vi "Service Mode Entry.vi"(0 "GEA2 Reference In":refnum<k24>, 5 "Model":enum16{"HE", "LE"}(ring), 11 "Error In":errorcluster) -> (4 "GEA2 Reference Out":refnum<k24>, 6 "Pass/Fail?":bool, 8 "Report Text":string, 15 "Error Out":errorcluster)   [LabVIEW 2016, in "2015 VA Washer.lvlib"]
doc: "Use this VI to enter service mode."
uses:
  Projects/2015 VA Washer.lvlib
  C:/Automation/DLLs/PC Dot Net/GeaCommunication.dll
  Common/LabVIEW GEA2 Toolkit/LabVIEW_GEA2_Toolkit.lvlibp/type defs/Source_Destination.ctl
  Common/LabVIEW GEA2 Toolkit/LabVIEW_GEA2_Toolkit.lvlibp/type defs/ERD Read Data In.ctl
  Common/LabVIEW GEA2 Toolkit/LabVIEW_GEA2_Toolkit.lvlibp/type defs/Data Type.ctl
  type defs/Encoder Position.ctl
  Common/LabVIEW GEA2 Toolkit/LabVIEW_GEA2_Toolkit.lvlibp/type defs/ERD Write Data In.ctl
  Common/LabVIEW GEA2 Toolkit/LabVIEW_GEA2_Toolkit.lvlibp
panel:
  in  "Standalone?":bool
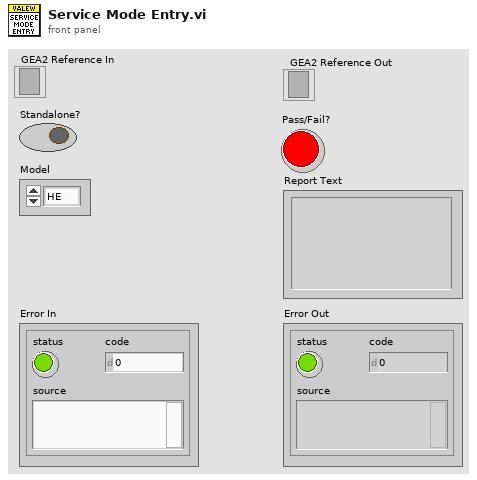
[diagram p1: front panel]
types:
  T1 = typedef "LabVIEW_GEA2_Toolkit.lvlibp/ERD Read Data In.ctl" = cluster{"ERD Number":u16, "Data Type":T2}
  T2 = typedef "LabVIEW_GEA2_Toolkit.lvlibp/Data Type.ctl" = enum16{"string", "boolean", "uint8_t", "uint16_t", "uint32_t", "uint64_t", "int8_t", "int16_t", "int32_t", "int64_t"}
  T3 = typedef "LabVIEW_GEA2_Toolkit.lvlibp/Source_Destination.ctl" = cluster{"Source":u8, "Destination":u8}
  T4 = typedef "LabVIEW_GEA2_Toolkit.lvlibp/ERD Write Data In.ctl" = cluster{"ERD Number":u16, "Data Type":T2, "Data":string}
  T5 = typedef "2015 VA Washer.lvlib/Encoder Position.ctl" = enum16{"Position 0", "Position 1", "Position 2", "Position 3", "Position 4", "Position 5", "Position 6", "Position 7", "Position 8", "Position 9", "Position 10", "Position 11", "Position 12", "Position 13", "Clear / Reset"}
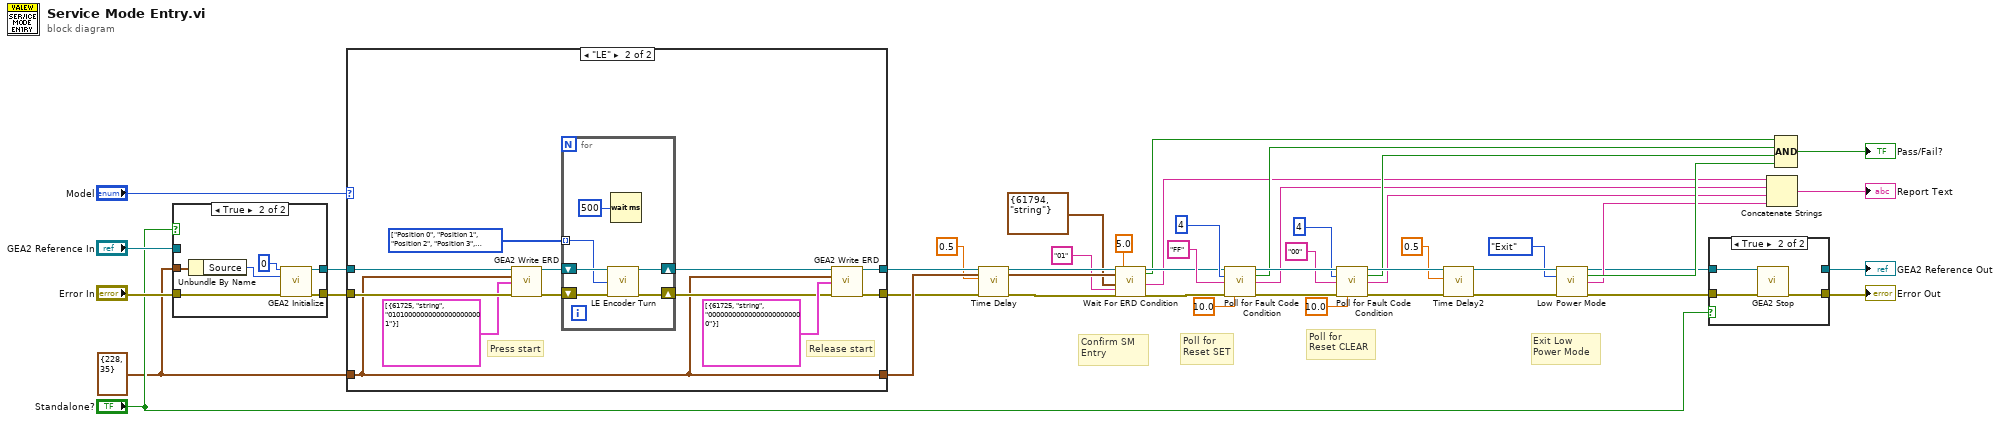
[diagram p0: block diagram]
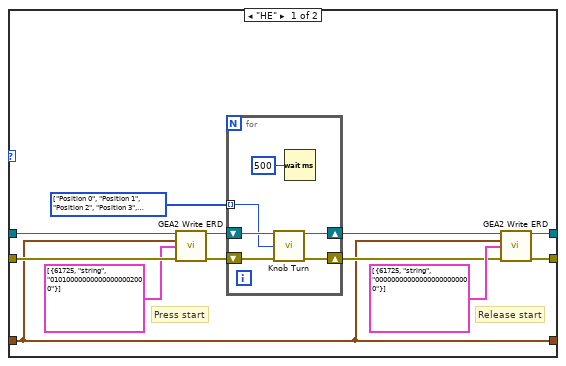
[diagram p2: hidden frame]
diagram:
  w37 = T3 {"Source"=228, "Destination"=35} ("GEA Inputs")
  # "Confirm SM \nEntry"
  # "Exit Low \nPower Mode"
  # "Poll for\nReset CLEAR"
  # "Poll for\nReset SET"
  n1 = case shown="True" "Standalone?" {
    tunnel: "Error In" -> [w45 w52]
    tunnel: [w45 w51] -> w39
    tunnel: "GEA2 Reference In" -> [w46 _]
    tunnel: [w46 w50] -> w40
    tunnel: w37 -> [_ w48]
    frame False {
    }
    frame True {
      n2 = Unbundle By Name(w48) -> ("Source"=w49:u8)
      n3 = call "GEA2 Initialize.vi"("Board Index"=0, "Source Address"=w49, "error in"=w52) -> ("GEA2 Reference Out"=w50:refnum<k24>, "error out"=w51:errorcluster)  [unwired: 10 in, 1 out]
    }
  }
  n4 = case shown="\"LE\"" "Model" {
    tunnel: w40 -> [w61 w79]
    tunnel: w39 -> [w60 w78]
    tunnel: w37 -> [w53 w71]
    tunnel: [w55 w73] -> w36
    tunnel: [w54 w72] -> w34
    tunnel: [w53 w71] -> w35
    frame "HE" {
      w64 = T5[] [enum."Position 0", enum."Position 1", enum."Position 2", enum."Position 3", enum."Position 4", enum."Position 5", enum."Position 6", enum."Position 7"] items=["Position 0", "Position 1", "Position 2", "Position 3", "Position 4", "Position 5", "Position 6", "Position 7", "Position 8", "Position 9", "Position 10", "Position 11", "Position 12", "Position 13", "Clear / Reset"]
      # "Release start"
      # "Press start"
      n5 = call "GEA2 Write ERD.vi"("GEA2 Reference In"=w61, "GEA Inputs"=w53, "Write ERD List"=T4[] [{"ERD Number"=61725, "Data Type"=enum."string", "Data"="010100000000000000002000"}], "Error In"=w60) -> ("GEA2 Reference Out"=w63:refnum<k24>, "Error Out"=w62:errorcluster)  [unwired: 9 in, 1 out]
      n6 = for {
        shift-right: [w69] -> w56
        shift-left: w63 -> [w70]
        shift-right: [w67] -> w57
        shift-left: w62 -> [w68]
        tunnel: w64 -> [w66] mode=indexing
        n7 = call "Knob Turn.vi"("GEA2 Reference In"=w70, "Button"=w66, "Error In"=w68) -> ("GEA2 Reference Out"=w69:refnum<k24>, "Error Out"=w67:errorcluster)  [unwired: 11 in]
        n8 = Wait (ms)(milliseconds to wait=u32 500) -> ()  [unwired: 1 out]
      }
      n9 = call "GEA2 Write ERD.vi"("GEA2 Reference In"=w56, "GEA Inputs"=w53, "Write ERD List"=T4[] [{"ERD Number"=61725, "Data Type"=enum."string", "Data"="000000000000000000000000"}], "Error In"=w57) -> ("GEA2 Reference Out"=w55:refnum<k24>, "Error Out"=w54:errorcluster)  [unwired: 9 in, 1 out]
    }
    frame "LE" {
      w82 = T5[] [enum."Position 0", enum."Position 1", enum."Position 2", enum."Position 3", enum."Position 4", enum."Position 5", enum."Position 6", enum."Position 7"] items=["Position 0", "Position 1", "Position 2", "Position 3", "Position 4", "Position 5", "Position 6", "Position 7", "Position 8", "Position 9", "Position 10", "Position 11", "Position 12", "Position 13", "Clear / Reset"]
      # "Release start"
      # "Press start"
      n10 = call "GEA2 Write ERD.vi"("GEA2 Reference In"=w79, "GEA Inputs"=w71, "Write ERD List"=T4[] [{"ERD Number"=61725, "Data Type"=enum."string", "Data"="010100000000000000000001"}], "Error In"=w78) -> ("GEA2 Reference Out"=w81:refnum<k24>, "Error Out"=w80:errorcluster)  [unwired: 9 in, 1 out]
      n11 = for {
        shift-right: [w87] -> w74
        shift-left: w81 -> [w88]
        shift-right: [w85] -> w75
        shift-left: w80 -> [w86]
        tunnel: w82 -> [w84] mode=indexing
        n12 = call "LE Encoder Turn.vi"("GEA2 Reference In"=w88, "Button"=w84, "Error In"=w86) -> ("GEA2 Reference Out"=w87:refnum<k24>, "Error Out"=w85:errorcluster)  [unwired: 11 in]
        n13 = Wait (ms)(milliseconds to wait=u32 500) -> ()  [unwired: 1 out]
      }
      n14 = call "GEA2 Write ERD.vi"("GEA2 Reference In"=w74, "GEA Inputs"=w71, "Write ERD List"=T4[] [{"ERD Number"=61725, "Data Type"=enum."string", "Data"="000000000000000000000000"}], "Error In"=w75) -> ("GEA2 Reference Out"=w73:refnum<k24>, "Error Out"=w72:errorcluster)  [unwired: 9 in, 1 out]
    }
  }
  n15 = call "Time Delay"("error in (no error)"=w34, "Delay Time (s)"=0.5) -> ("error out"=w5:errorcluster)  [unwired: 9 in]
  n16 = call "Wait For ERD Condition.vi"("GEA2 Reference In"=w36, "GEA Inputs"=w35, "ERD Read Data"=T1 {"ERD Number"=61794, "Data Type"=enum."string"} ("ERD Read Data In"), "Expected Low"="01", "Error In"=w5, "Timeout (s)"=5.0) -> ("GEA2 Reference Out"=w18:refnum<k24>, "Pass/Fail?"=w6:bool, "Report Text"=w7:string, "Error Out"=w20:errorcluster)  [unwired: 9 in, 1 out]
  n17 = call "Poll for Fault Code Condition.vi"("GEA2 Reference In"=w18, "Fault ID (Decimal)"=u16 4, "Fault Status (00/FF)"="FF", "Error In"=w20, "Timeout (s)"=10.0) -> ("GEA2 Reference Out"=w28:refnum<k24>, "Pass/Fail?"=w15:bool, "Report Text"=w14:string, "Error Out"=w29:errorcluster)  [unwired: 6 in, 1 out]
  n18 = call "Poll for Fault Code Condition.vi"("GEA2 Reference In"=w28, "Fault ID (Decimal)"=u16 4, "Fault Status (00/FF)"="00", "Error In"=w29, "Timeout (s)"=10.0) -> ("GEA2 Reference Out"=w26:refnum<k24>, "Pass/Fail?"=w16:bool, "Report Text"=w13:string, "Error Out"=w2:errorcluster)  [unwired: 6 in, 1 out]
  n19 = call "Time Delay2"("error in (no error)"=w2, "Delay Time (s)"=0.5) -> ("error out"=w1:errorcluster)  [unwired: 9 in]
  n20 = call "Low Power Mode.vi"("GEA2 Reference In"=w26, "Action"=enum16{"Enter", "Exit"}."Exit", "Error In"=w1) -> ("GEA2 Reference Out"=w9:refnum<k24>, "Pass/Fail?"=w17:bool, "Report Text"=w12:string, "Error Out"=w19:errorcluster)  [unwired: 9 in]
  n21 = case shown="True" "Standalone?" {
    tunnel: [w90 w93] -> w44
    tunnel: w19 -> [w90 w92]
    tunnel: w9 -> [w89 w91]
    tunnel: [w89 _] -> w8
    frame False {
    }
    frame True {
      n22 = call "GEA2 Stop.vi"("GEA2 Reference In"=w91, "Error In"=w92) -> ("Error Out"=w93:errorcluster)  [unwired: 13 in]
    }
  }
  "Error Out" <- w44
  "GEA2 Reference Out" <- w8
  n23 = Concatenate Strings(w7, w14, w13, w12) -> (→"Report Text":string)
  n24 = Compound Arithmetic op=AND(w6, w15, w16, w17) -> (→"Pass/Fail?":bool)
